vi "SetDIWord.vi"(2 "error in (no error)":errorcluster, 3 "DIDWord (obs)":bool, 4 "DIWord":bool, 5 "task in":refnum<k24>) -> (0 "error out":errorcluster, 1 "task out":refnum<k24>)   [LabVIEW 2010]
uses:
  C:/Program Files/National Instruments/LabVIEW 2010/vi.lib/ULx/ULx_LV.dll
  Program Files/National Instruments/LabVIEW 2010/vi.lib/ULx/ULx_LV.dll
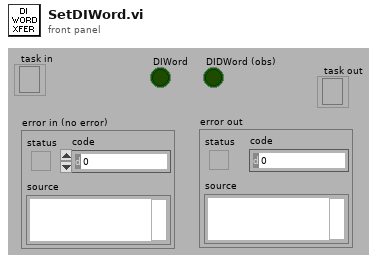
[diagram p1: front panel]
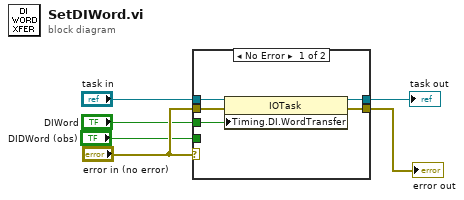
[diagram p0: block diagram]
diagram:
  n1 = case shown="No Error" "error in (no error)" {
    tunnel: "task in" -> [w11 w13]
    tunnel: "error in (no error)" -> [w10 w12]
    tunnel: [w9 w13] -> w5
    tunnel: [w8 w12] -> w4
    tunnel: "DIWord" -> [w7 _]
    tunnel: "DIDWord (obs)" -> [_ _]
    frame No Error {
      n2 = property class="IOTask"(reference=w11, error in=w10, "Timing.DI.WordTransfer"=w7) -> (reference out=w9:refnum<k24>, error out=w8:errorcluster)
    }
    frame Error {
    }
  }
  "task out" <- w5
  "error out" <- w4
